vi "TempoAtual.vi"(11 "TimeInicio":u32) -> (3 "TempoAtual":dbl)   [LabVIEW 2019]
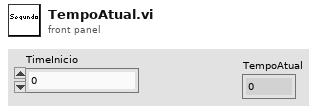
[diagram p1: front panel]
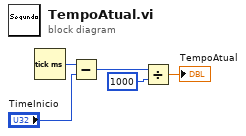
[diagram p0: block diagram]
diagram:
  n1 = Tick Count (ms)() -> (millisecond timer value=w4:u32)
  n2 = Subtract(x=w4, y="TimeInicio") -> (x-y=w5:u32)
  n3 = Divide(x=w5, y=u32 1000) -> (x/y=→"TempoAtual":dbl)
